vi "Run.vi"(8 "error in (no error)":errorcluster, 11 "Application in":refnum<class "Application.lvclass">) -> (0 "error out":errorcluster, 3 "Application out":refnum<class "Application.lvclass">)   [LabVIEW 2018, in "Application.lvclass"]
doc: "Este VI realiza a comunicação com as cãmeras através de uma estrutura de Fila. Possui uma máquina de estados que realiza o gerenciamento de cada informação que deve ser mandada para as câmeras e, também, é responsável por retornar o gráfico da última imagem obtida."
uses:
  Application.lvclass
  Application.lvclass/Application.ctl
  Instrument/Instrument.lvclass/Instrument.ctl
  State Machine/State Machine.lvclass/State Machine.ctl
  RxTx/RxTx.lvclass/RxTx.ctl
  CCDCamera/CCDCamera.lvclass/CCDCamera.ctl
  RxTXCamera/RxTxCamera.lvclass/RxTxCamera.ctl
  Construct String Header/Construct String Header.lvclass/Construct String Header.ctl
  RxTx/Write Message.vi
  RxTXCamera/Write Construct String Header.lvclass.vi
  RxTXCamera/Read Construct String Header.lvclass.vi
  Construct String Header/Write Header Contents.vi
  CCDCamera/CCDCamera.lvclass
  C:/Users/Cliente/Desktop/Software Echarpe/Instrument/Instrument.lvclass
  RxTXCamera/RxTxCamera.lvclass
  C:/Users/Cliente/Desktop/Software Echarpe/RxTx/RxTx.lvclass
  Construct String Header/Make string.vi
  State Machine/State Machine.lvclass
  Construct String Header/Construct String Header.lvclass
  Display Image/Display Image.lvclass
  Instrument/Instrument.lvclass
  RxTx/RxTx.lvclass
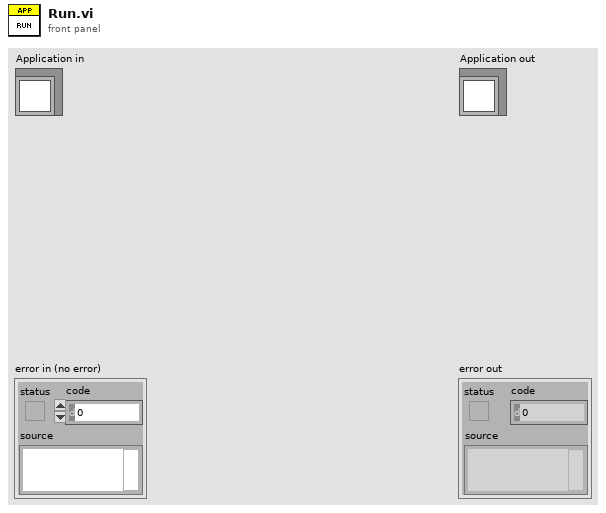
[diagram p1: front panel]
types:
  T1 = cluster{"Currently Temperature":dbl, "Last Image":string, "% Acquired":dbl, "Initilizarion":bool, "Exposing":bool, "Temperature Status":string, "X length":dbl, "Y length":dbl, "Min Temperature":dbl, "Max Temperature":dbl}
  T2 = cluster{"FILENAME":string[], "OBSERVER":string[], "PROGRID":string[], "OBJECT":string[], "NIGHTDIR":string[], "CHANNEL":string[], "INSTRUME":string[], "NEXPSEQ":string[], "SEQINDEX":string[], "OBSTYPE":string[], "READMOD":string[], "SHUTTER":string[], "OPENSHT":string[], "CLOSESHT":string[], "GAIN":string[], "GAINERR ":string[], "RDNOISE":string[], "RNOISERR":string[], "SKYFIBER":string[], "CALFIBER":string[], "UTDATE":string[], "LOCTIME":string[], "MJD":string[], "OBSLON":string[], "OBSLAT":string[], "OBSALT":string[], "EXPTIME":string[], "TELRA":string[], "TELDEC":string[], "RA":string[], "DEC":string[], "RA_DEG":string[], "DEC_DEG":string[], "EPOCH":string[], "HA":string[], "HAD":string[], "AIRMASS":string[], "AMSTART":string[], "AMEND":string[], "XOFFSET":string[], "YOFFSET":string[], "PA":string[], "CAMFOC":string[], "TELFOC":string[], "TCSUT":string[], "MOONDIST":string[], "MOONALT":string[], "MONNPHAS":string[], "ADC":string[], "ADCSPPED":string[], "CALMIRR":string[], "GUIDING":string[], "GUIDTEXP":string[], "GUIDFREQ":string[], "GUIDOBJX":string[], "GUIDOBJY":string[], "AVGYCORR":string[], "AVGXCORR":string[], "GFOCUS":string[], "THARLAMP":string[], "HALLAMP":string[], "AGITATOR":string[], "THARMIRR":string[], "DSTATUS":string[], "DTEMP":string[], "DHUM":string[], "DLAMP":string[], "DFLAT":string[], "TEMPEXT":string[], "PRESSURE":string[], "HUMIDITY":string[], "WINDDIR":string[], "WSPEED":string[], "TCSST":string[], "DPOS":string[]}
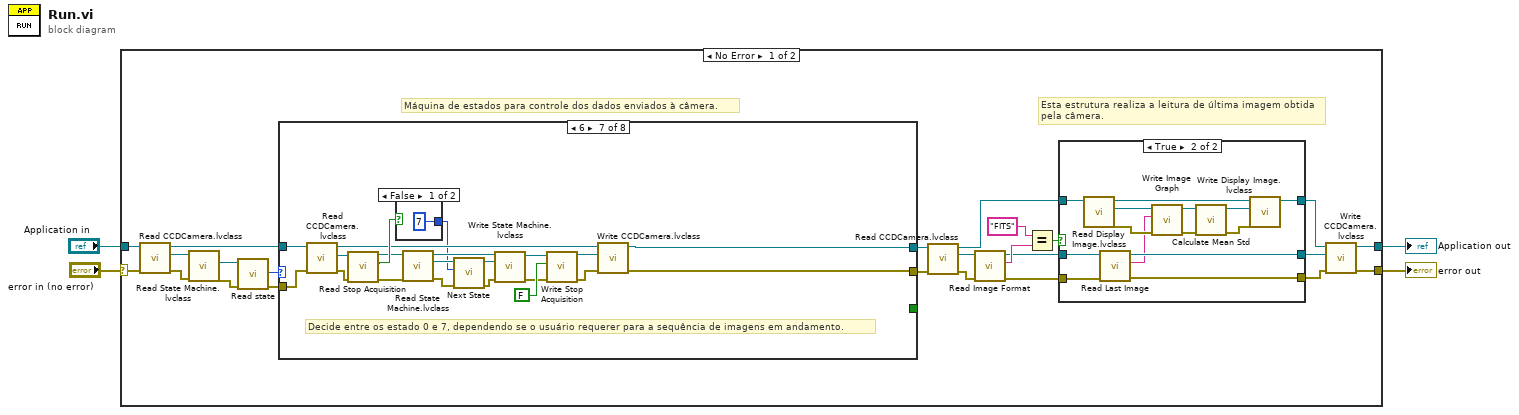
[diagram p0: block diagram]
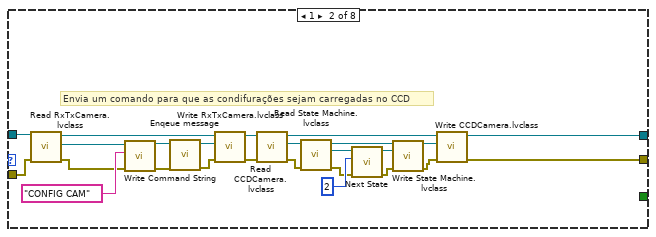
[diagram p3: hidden frame]
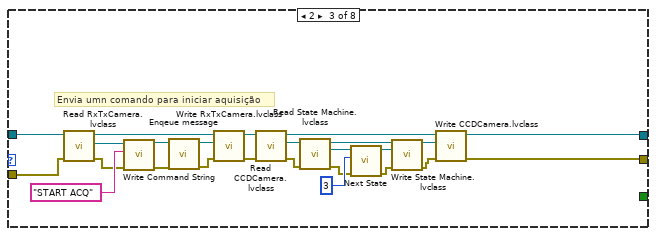
[diagram p4: hidden frame]
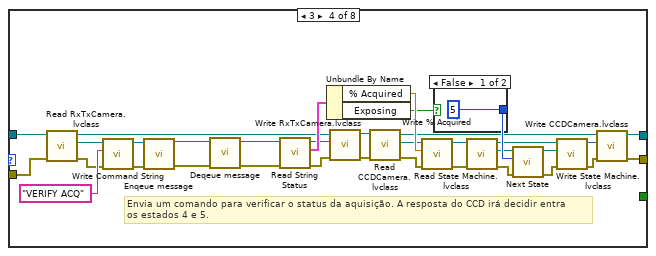
[diagram p5: hidden frame]
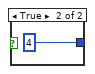
[diagram p6: hidden frame]
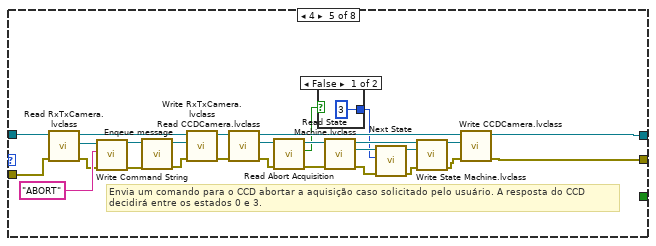
[diagram p7: hidden frame]
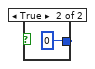
[diagram p8: hidden frame]
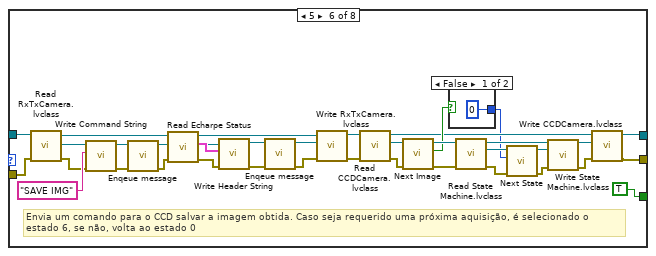
[diagram p9: hidden frame]
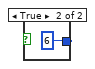
[diagram p10: hidden frame]
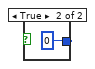
[diagram p11: hidden frame]
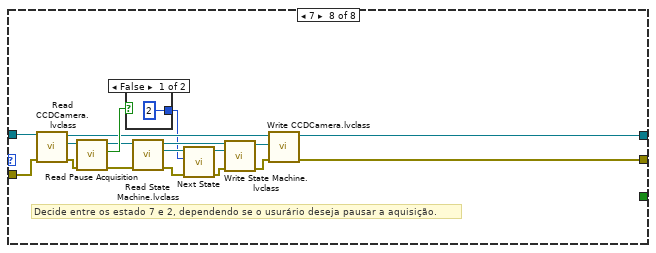
[diagram p12: hidden frame]
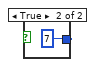
[diagram p13: hidden frame]
diagram:
  n1 = case shown="No Error" "error in (no error)" {
    selector: "error in (no error)" -> [w27 w246]
    tunnel: [w21 w246] -> w3
    tunnel: [w22 w245] -> w1
    tunnel: "Application in" -> [w28 w245]
    frame No Error {
      # "Esta estrutura realiza a leitura de última imagem obtida\npela câmera."
      # "Máquina de estados para controle dos dados enviados à câmera."
      n2 = call "Read CCDCamera.lvclass.vi"("error in (no error)"=w27, "Application in"=w28) -> ("error out"=w25:errorcluster, "CCDCamera.lvclass"=w26:refnum<class "CCDCamera.lvclass">, "Application out"=w7:refnum<class "Application.lvclass">)  [unwired: 7 in]
      n3 = call "Read State Machine.lvclass.vi"("error in (no error)"=w25, "Instrument in"=w26) -> ("error out"=w23:errorcluster, "State Machine.lvclass"=w24:refnum<class "State Machine.lvclass">)  [unwired: 7 in, 1 out]
      n4 = call "Read state.vi"("error in (no error)"=w23, "State Machine in"=w24) -> ("error out"=w6:errorcluster, "state"=w5:u32)  [unwired: 7 in, 1 out]
      n5 = case shown="6" w5 {
        tunnel: w6 -> [w29 w55 w58 w113 w125 w154 w187 w210]
        tunnel: w7 -> [w30 w54 w59 w114 w126 w155 w188 w211]
        tunnel: [w30 w32 w57 w82 w118 w168 w185 w209] -> w8
        tunnel: [w29 w31 w56 w81 w117 w167 w186 w208] -> w9
        tunnel: [_ _ _ _ _ TRUE _ _] -> _
        frame 0, Default {
        }
        frame 1 {
          # "Envia um comando para que as condifurações sejam carregadas no CCD"
          n6 = call "Read RxTxCamera.lvclass.vi"("error in (no error)"=w55, "Application in"=w54) -> ("error out"=w46:errorcluster, "RxTxCamera.lvclass"=w48:refnum<class "RxTxCamera.lvclass">, "Application out"=w52:refnum<class "Application.lvclass">)  [unwired: 7 in]
          n7 = call "Write Command String.vi"("error in (no error)"=w46, "Command String"="CONFIG CAM", "RxTxCamera in"=w48) -> ("error out"=w51:errorcluster, "RxTxCamera out"=w50:refnum<class "RxTxCamera.lvclass">)  [unwired: 7 in]
          n8 = call "Enqeue message.vi"("error in (no error)"=w51, "RxTx in"=w50) -> ("error out"=w53:errorcluster, "RxTx out"=w49:refnum<class "RxTxCamera.lvclass">)  [unwired: 8 in]
          n9 = call "Write RxTxCamera.lvclass.vi"("error in (no error)"=w53, "RxTxCamera.lvclass"=w49, "Application in"=w52) -> ("error out"=w45:errorcluster, "Application out"=w44:refnum<class "Application.lvclass">)  [unwired: 7 in]
          n10 = call "Read CCDCamera.lvclass.vi"("error in (no error)"=w45, "Application in"=w44) -> ("error out"=w43:errorcluster, "CCDCamera.lvclass"=w42:refnum<class "CCDCamera.lvclass">, "Application out"=w35:refnum<class "Application.lvclass">)  [unwired: 7 in]
          n11 = call "Read State Machine.lvclass.vi"("error in (no error)"=w43, "Instrument in"=w42) -> ("error out"=w40:errorcluster, "State Machine.lvclass"=w39:refnum<class "State Machine.lvclass">, "Instrument out"=w36:refnum<class "CCDCamera.lvclass">)  [unwired: 7 in]
          n12 = call "Next State.vi"("error in (no error)"=w40, "New_State"=u32 2, "State Machine in"=w39) -> ("error out"=w38:errorcluster, "State Machine out"=w37:refnum<class "State Machine.lvclass">)  [unwired: 7 in]
          n13 = call "Write State Machine.lvclass.vi"("error in (no error)"=w38, "State Machine.lvclass"=w37, "Instrument in"=w36) -> ("error out"=w34:errorcluster, "Instrument out"=w33:refnum<class "CCDCamera.lvclass">)  [unwired: 7 in]
          n14 = call "Write CCDCamera.lvclass.vi"("error in (no error)"=w34, "CCDCamera.lvclass"=w33, "Application in"=w35) -> ("error out"=w31:errorcluster, "Application out"=w32:refnum<class "Application.lvclass">)  [unwired: 7 in]
        }
        frame 2 {
          # "Envia umn comando para iniciar aquisição"
          n15 = call "Read RxTxCamera.lvclass.vi"("error in (no error)"=w58, "Application in"=w59) -> ("error out"=w73:errorcluster, "RxTxCamera.lvclass"=w75:refnum<class "RxTxCamera.lvclass">, "Application out"=w79:refnum<class "Application.lvclass">)  [unwired: 7 in]
          n16 = call "Write Command String.vi"("error in (no error)"=w73, "Command String"="START ACQ", "RxTxCamera in"=w75) -> ("error out"=w78:errorcluster, "RxTxCamera out"=w77:refnum<class "RxTxCamera.lvclass">)  [unwired: 7 in]
          n17 = call "Enqeue message.vi"("error in (no error)"=w78, "RxTx in"=w77) -> ("error out"=w80:errorcluster, "RxTx out"=w76:refnum<class "RxTxCamera.lvclass">)  [unwired: 8 in]
          n18 = call "Write RxTxCamera.lvclass.vi"("error in (no error)"=w80, "RxTxCamera.lvclass"=w76, "Application in"=w79) -> ("error out"=w72:errorcluster, "Application out"=w71:refnum<class "Application.lvclass">)  [unwired: 7 in]
          n19 = call "Read CCDCamera.lvclass.vi"("error in (no error)"=w72, "Application in"=w71) -> ("error out"=w70:errorcluster, "CCDCamera.lvclass"=w69:refnum<class "CCDCamera.lvclass">, "Application out"=w62:refnum<class "Application.lvclass">)  [unwired: 7 in]
          n20 = call "Read State Machine.lvclass.vi"("error in (no error)"=w70, "Instrument in"=w69) -> ("error out"=w67:errorcluster, "State Machine.lvclass"=w66:refnum<class "State Machine.lvclass">, "Instrument out"=w63:refnum<class "CCDCamera.lvclass">)  [unwired: 7 in]
          n21 = call "Next State.vi"("error in (no error)"=w67, "New_State"=u32 3, "State Machine in"=w66) -> ("error out"=w65:errorcluster, "State Machine out"=w64:refnum<class "State Machine.lvclass">)  [unwired: 7 in]
          n22 = call "Write State Machine.lvclass.vi"("error in (no error)"=w65, "State Machine.lvclass"=w64, "Instrument in"=w63) -> ("error out"=w61:errorcluster, "Instrument out"=w60:refnum<class "CCDCamera.lvclass">)  [unwired: 7 in]
          n23 = call "Write CCDCamera.lvclass.vi"("error in (no error)"=w61, "CCDCamera.lvclass"=w60, "Application in"=w62) -> ("error out"=w56:errorcluster, "Application out"=w57:refnum<class "Application.lvclass">)  [unwired: 7 in]
        }
        frame 3 {
          # "Envia um comando para verificar o status da aquisição. A resposta do CCD irá decidir entra\nos estados 4 e 5."
          n24 = call "Read RxTxCamera.lvclass.vi"("error in (no error)"=w113, "Application in"=w114) -> ("error out"=w106:errorcluster, "RxTxCamera.lvclass"=w107:refnum<class "RxTxCamera.lvclass">, "Application out"=w100:refnum<class "Application.lvclass">)  [unwired: 7 in]
          n25 = call "Write Command String.vi"("error in (no error)"=w106, "Command String"="VERIFY ACQ", "RxTxCamera in"=w107) -> ("error out"=w109:errorcluster, "RxTxCamera out"=w105:refnum<class "RxTxCamera.lvclass">)  [unwired: 7 in]
          n26 = call "Enqeue message.vi"("error in (no error)"=w109, "RxTx in"=w105) -> ("error out"=w104:errorcluster, "RxTx out"=w103:refnum<class "RxTxCamera.lvclass">)  [unwired: 8 in]
          n27 = call "Deqeue message.vi"("error in (no error)"=w104, "RxTx in"=w103) -> ("error out"=w112:errorcluster, "RxTx out"=w111:refnum<class "RxTxCamera.lvclass">)  [unwired: 8 in]
          n28 = call "Read String Status.vi"("error in (no error)"=w112, "RxTxCamera in"=w111) -> ("error out"=w102:errorcluster, "Camera Status"=w110:T1, "RxTxCamera out"=w101:refnum<class "RxTxCamera.lvclass">)  [unwired: 7 in]
          n29 = Unbundle By Name(w110) -> ("% Acquired"=w97:dbl, "Exposing"=w90:bool)
          n30 = call "Write RxTxCamera.lvclass.vi"("error in (no error)"=w102, "RxTxCamera.lvclass"=w101, "Application in"=w100) -> ("error out"=w99:errorcluster, "Application out"=w98:refnum<class "Application.lvclass">)  [unwired: 7 in]
          n31 = call "Read CCDCamera.lvclass.vi"("error in (no error)"=w99, "Application in"=w98) -> ("error out"=w95:errorcluster, "CCDCamera.lvclass"=w96:refnum<class "CCDCamera.lvclass">, "Application out"=w83:refnum<class "Application.lvclass">)  [unwired: 7 in]
          n32 = call "Write % Acquired.vi"("error in (no error)"=w95, "% Acquired"=w97, "CCDCamera in"=w96) -> ("error out"=w92:errorcluster, "CCDCamera out"=w91:refnum<class "CCDCamera.lvclass">)  [unwired: 7 in]
          n33 = case shown="False" w90 {
            tunnel: [u32 5 ("New_State") u32 4 ("New_State")] -> w89
            frame False {
            }
            frame True {
            }
          }
          n34 = call "Read State Machine.lvclass.vi"("error in (no error)"=w92, "Instrument in"=w91) -> ("error out"=w94:errorcluster, "State Machine.lvclass"=w88:refnum<class "State Machine.lvclass">, "Instrument out"=w86:refnum<class "CCDCamera.lvclass">)  [unwired: 7 in]
          n35 = call "Next State.vi"("error in (no error)"=w94, "New_State"=w89, "State Machine in"=w88) -> ("error out"=w93:errorcluster, "State Machine out"=w87:refnum<class "State Machine.lvclass">)  [unwired: 7 in]
          n36 = call "Write State Machine.lvclass.vi"("error in (no error)"=w93, "State Machine.lvclass"=w87, "Instrument in"=w86) -> ("error out"=w85:errorcluster, "Instrument out"=w84:refnum<class "CCDCamera.lvclass">)  [unwired: 7 in]
          n37 = call "Write CCDCamera.lvclass.vi"("error in (no error)"=w85, "CCDCamera.lvclass"=w84, "Application in"=w83) -> ("error out"=w81:errorcluster, "Application out"=w82:refnum<class "Application.lvclass">)  [unwired: 7 in]
        }
        frame 4 {
          # "Envia um comando para o CCD abortar a aquisição caso solicitado pelo usuário. A resposta do CCD\ndecidirá entre os estados 0 e 3."
          n38 = call "Read RxTxCamera.lvclass.vi"("error in (no error)"=w125, "Application in"=w126) -> ("error out"=w137:errorcluster, "RxTxCamera.lvclass"=w139:refnum<class "RxTxCamera.lvclass">, "Application out"=w143:refnum<class "Application.lvclass">)  [unwired: 7 in]
          n39 = call "Write Command String.vi"("error in (no error)"=w137, "Command String"="ABORT", "RxTxCamera in"=w139) -> ("error out"=w142:errorcluster, "RxTxCamera out"=w141:refnum<class "RxTxCamera.lvclass">)  [unwired: 7 in]
          n40 = call "Enqeue message.vi"("error in (no error)"=w142, "RxTx in"=w141) -> ("error out"=w144:errorcluster, "RxTx out"=w140:refnum<class "RxTxCamera.lvclass">)  [unwired: 8 in]
          n41 = call "Write RxTxCamera.lvclass.vi"("error in (no error)"=w144, "RxTxCamera.lvclass"=w140, "Application in"=w143) -> ("error out"=w136:errorcluster, "Application out"=w135:refnum<class "Application.lvclass">)  [unwired: 7 in]
          n42 = call "Read CCDCamera.lvclass.vi"("error in (no error)"=w136, "Application in"=w135) -> ("error out"=w123:errorcluster, "CCDCamera.lvclass"=w124:refnum<class "CCDCamera.lvclass">, "Application out"=w129:refnum<class "Application.lvclass">)  [unwired: 7 in]
          n43 = call "Read Abort Acquisition.vi"("error in (no error)"=w123, "CCDCamera in"=w124) -> ("error out"=w122:errorcluster, "Abort Acquisition"=w120:bool, "CCDCamera out"=w121:refnum<class "CCDCamera.lvclass">)  [unwired: 7 in]
          n44 = case shown="False" w120 {
            tunnel: [u32 3 ("New_State") u32 0 ("New_State")] -> w119
            frame False {
            }
            frame True {
            }
          }
          n45 = call "Read State Machine.lvclass.vi"("error in (no error)"=w122, "Instrument in"=w121) -> ("error out"=w134:errorcluster, "State Machine.lvclass"=w133:refnum<class "State Machine.lvclass">, "Instrument out"=w130:refnum<class "CCDCamera.lvclass">)  [unwired: 7 in]
          n46 = call "Next State.vi"("error in (no error)"=w134, "New_State"=w119, "State Machine in"=w133) -> ("error out"=w132:errorcluster, "State Machine out"=w131:refnum<class "State Machine.lvclass">)  [unwired: 7 in]
          n47 = call "Write State Machine.lvclass.vi"("error in (no error)"=w132, "State Machine.lvclass"=w131, "Instrument in"=w130) -> ("error out"=w128:errorcluster, "Instrument out"=w127:refnum<class "CCDCamera.lvclass">)  [unwired: 7 in]
          n48 = call "Write CCDCamera.lvclass.vi"("error in (no error)"=w128, "CCDCamera.lvclass"=w127, "Application in"=w129) -> ("error out"=w117:errorcluster, "Application out"=w118:refnum<class "Application.lvclass">)  [unwired: 7 in]
        }
        frame 5 {
          # "Envia um comando para o CCD salvar a imagem obtida. Caso seja requerido uma próxima aquisição, é selecionado o \nestado 6, se não, volta ao estado 0"
          n49 = call "Read RxTxCamera.lvclass.vi"("error in (no error)"=w154, "Application in"=w155) -> ("error out"=w152:errorcluster, "RxTxCamera.lvclass"=w151:refnum<class "RxTxCamera.lvclass">, "Application out"=w159:refnum<class "Application.lvclass">)  [unwired: 7 in]
          n50 = call "Write Command String.vi"("error in (no error)"=w152, "Command String"="SAVE IMG", "RxTxCamera in"=w151) -> ("error out"=w150:errorcluster, "RxTxCamera out"=w148:refnum<class "RxTxCamera.lvclass">)  [unwired: 7 in]
          n51 = call "Enqeue message.vi"("error in (no error)"=w150, "RxTx in"=w148) -> ("error out"=w149:errorcluster, "RxTx out"=w147:refnum<class "RxTxCamera.lvclass">)  [unwired: 8 in]
          n52 = call "Read Echarpe Status.vi"("error in (no error)"=w149, "Application in"=w159) -> ("error out"=w162:errorcluster, "Header Contents out"=w161:T2, "Application out"=w160:refnum<class "Application.lvclass">)  [unwired: 7 in]
          n53 = call "Write Header String.vi"("error in (no error)"=w162, "Header Contents"=w161, "RxTxCamera in"=w147) -> ("error out"=w163:errorcluster, "RxTxCamera out"=w164:refnum<class "RxTxCamera.lvclass">)  [unwired: 7 in]
          n54 = call "Enqeue message.vi"("error in (no error)"=w163, "RxTx in"=w164) -> ("error out"=w165:errorcluster, "RxTx out"=w166:refnum<class "RxTxCamera.lvclass">)  [unwired: 8 in]
          n55 = call "Write RxTxCamera.lvclass.vi"("error in (no error)"=w165, "RxTxCamera.lvclass"=w166, "Application in"=w160) -> ("error out"=w157:errorcluster, "Application out"=w156:refnum<class "Application.lvclass">)  [unwired: 7 in]
          n56 = call "Read CCDCamera.lvclass.vi"("error in (no error)"=w157, "Application in"=w156) -> ("error out"=w178:errorcluster, "CCDCamera.lvclass"=w179:refnum<class "CCDCamera.lvclass">, "Application out"=w172:refnum<class "Application.lvclass">)  [unwired: 7 in]
          n57 = call "Next Image"("error in (no error)"=w178, "CCDCamera in"=w179) -> ("error out"=w182:errorcluster, "Next Image ?"=w180:bool, "CCDCamera out"=w181:refnum<class "CCDCamera.lvclass">)  [unwired: 7 in]
          n58 = case shown="False" w180 {
            tunnel: [u32 0 ("New_State") u32 6 ("New_State")] -> w169
            frame False {
            }
            frame True {
            }
          }
          n59 = call "Read State Machine.lvclass.vi"("error in (no error)"=w182, "Instrument in"=w181) -> ("error out"=w177:errorcluster, "State Machine.lvclass"=w176:refnum<class "State Machine.lvclass">, "Instrument out"=w173:refnum<class "CCDCamera.lvclass">)  [unwired: 7 in]
          n60 = call "Next State.vi"("error in (no error)"=w177, "New_State"=w169, "State Machine in"=w176) -> ("error out"=w175:errorcluster, "State Machine out"=w174:refnum<class "State Machine.lvclass">)  [unwired: 7 in]
          n61 = call "Write State Machine.lvclass.vi"("error in (no error)"=w175, "State Machine.lvclass"=w174, "Instrument in"=w173) -> ("error out"=w171:errorcluster, "Instrument out"=w170:refnum<class "CCDCamera.lvclass">)  [unwired: 7 in]
          n62 = call "Write CCDCamera.lvclass.vi"("error in (no error)"=w171, "CCDCamera.lvclass"=w170, "Application in"=w172) -> ("error out"=w167:errorcluster, "Application out"=w168:refnum<class "Application.lvclass">)  [unwired: 7 in]
        }
        frame 6 {
          # "Decide entre os estado 0 e 7, dependendo se o usuário requerer para a sequência de imagens em andamento."
          n63 = call "Read CCDCamera.lvclass.vi"("error in (no error)"=w187, "Application in"=w188) -> ("error out"=w197:errorcluster, "CCDCamera.lvclass"=w196:refnum<class "CCDCamera.lvclass">, "Application out"=w190:refnum<class "Application.lvclass">)  [unwired: 7 in]
          n64 = call "Read Stop Acquisition.vi"("error in (no error)"=w197, "CCDCamera in"=w196) -> ("error out"=w198:errorcluster, "Stop Acquisition"=w200:bool, "CCDCamera out"=w199:refnum<class "CCDCamera.lvclass">)  [unwired: 7 in]
          n65 = case shown="False" w200 {
            tunnel: [u32 7 ("New_State") u32 0 ("New_State")] -> w189
            frame False {
            }
            frame True {
            }
          }
          n66 = call "Read State Machine.lvclass.vi"("error in (no error)"=w198, "Instrument in"=w199) -> ("error out"=w195:errorcluster, "State Machine.lvclass"=w194:refnum<class "State Machine.lvclass">, "Instrument out"=w191:refnum<class "CCDCamera.lvclass">)  [unwired: 7 in]
          n67 = call "Next State.vi"("error in (no error)"=w195, "New_State"=w189, "State Machine in"=w194) -> ("error out"=w193:errorcluster, "State Machine out"=w192:refnum<class "State Machine.lvclass">)  [unwired: 7 in]
          n68 = call "Write State Machine.lvclass.vi"("error in (no error)"=w193, "State Machine.lvclass"=w192, "Instrument in"=w191) -> ("error out"=w201:errorcluster, "Instrument out"=w202:refnum<class "CCDCamera.lvclass">)  [unwired: 7 in]
          n69 = call "Write Stop Acquisition.vi"("error in (no error)"=w201, "Stop Acquisition"=FALSE, "CCDCamera in"=w202) -> ("error out"=w203:errorcluster, "CCDCamera out"=w204:refnum<class "CCDCamera.lvclass">)  [unwired: 7 in]
          n70 = call "Write CCDCamera.lvclass.vi"("error in (no error)"=w203, "CCDCamera.lvclass"=w204, "Application in"=w190) -> ("error out"=w186:errorcluster, "Application out"=w185:refnum<class "Application.lvclass">)  [unwired: 7 in]
        }
        frame 7 {
          # "Decide entre os estado 7 e 2, dependendo se o usurário deseja pausar a aquisição."
          n71 = call "Read CCDCamera.lvclass.vi"("error in (no error)"=w210, "Application in"=w211) -> ("error out"=w219:errorcluster, "CCDCamera.lvclass"=w220:refnum<class "CCDCamera.lvclass">, "Application out"=w213:refnum<class "Application.lvclass">)  [unwired: 7 in]
          n72 = call "Read Pause Acquisition.vi"("error in (no error)"=w219, "CCDCamera in"=w220) -> ("error out"=w221:errorcluster, "Pause Acquisition"=w223:bool, "CCDCamera out"=w222:refnum<class "CCDCamera.lvclass">)  [unwired: 7 in]
          n73 = case shown="False" w223 {
            tunnel: [u32 2 ("New_State") u32 7 ("New_State")] -> w212
            frame False {
            }
            frame True {
            }
          }
          n74 = call "Read State Machine.lvclass.vi"("error in (no error)"=w221, "Instrument in"=w222) -> ("error out"=w218:errorcluster, "State Machine.lvclass"=w217:refnum<class "State Machine.lvclass">, "Instrument out"=w214:refnum<class "CCDCamera.lvclass">)  [unwired: 7 in]
          n75 = call "Next State.vi"("error in (no error)"=w218, "New_State"=w212, "State Machine in"=w217) -> ("error out"=w216:errorcluster, "State Machine out"=w215:refnum<class "State Machine.lvclass">)  [unwired: 7 in]
          n76 = call "Write State Machine.lvclass.vi"("error in (no error)"=w216, "State Machine.lvclass"=w215, "Instrument in"=w214) -> ("error out"=w224:errorcluster, "Instrument out"=w225:refnum<class "CCDCamera.lvclass">)  [unwired: 7 in]
          n77 = call "Write CCDCamera.lvclass.vi"("error in (no error)"=w224, "CCDCamera.lvclass"=w225, "Application in"=w213) -> ("error out"=w208:errorcluster, "Application out"=w209:refnum<class "Application.lvclass">)  [unwired: 7 in]
        }
      }
      n78 = call "Read CCDCamera.lvclass.vi"("error in (no error)"=w9, "Application in"=w8) -> ("error out"=w12:errorcluster, "CCDCamera.lvclass"=w11:refnum<class "CCDCamera.lvclass">, "Application out"=w10:refnum<class "Application.lvclass">)  [unwired: 7 in]
      n79 = call "Read Image Format.vi"("error in (no error)"=w12, "CCDCamera in"=w11) -> ("error out"=w13:errorcluster, "Image Format"=w16:string, "CCDCamera out"=w14:refnum<class "CCDCamera.lvclass">)  [unwired: 7 in]
      n80 = Equal?(x="FITS", y=w16) -> (x = y?=w17:bool)
      n81 = case shown="True" w17 {
        tunnel: [w228 w237] -> w20
        tunnel: [w230 w236] -> w19
        tunnel: [w229 w235] -> w18
        tunnel: w13 -> [w229 w234]
        tunnel: w14 -> [w230 w233]
        tunnel: w10 -> [w228 w231]
        frame False {
        }
        frame True {
          n82 = call "Read Display Image.lvclass.vi"("Application in"=w231) -> ("error out"=w243:errorcluster, "Display Image.lvclass"=w244:refnum<class "Display Image.lvclass">, "Application out"=w238:refnum<class "Application.lvclass">)  [unwired: 8 in]
          n83 = call "Read Last Image.vi"("error in (no error)"=w234, "CCDCamera in"=w233) -> ("error out"=w235:errorcluster, "Last Image Path"=w232:string, "CCDCamera out"=w236:refnum<class "CCDCamera.lvclass">)  [unwired: 6 in, 1 out]
          n84 = call "Write Image Graph.vi"("error in (no error)"=w243, "file path"=w232, "Display Image in"=w244) -> ("error out"=w242:errorcluster, "Display Image out"=w241:refnum<class "Display Image.lvclass">)  [unwired: 7 in]
          n85 = call "Calculate Mean Std.vi"("error in (no error)"=w242, "Display Image in"=w241) -> ("error out"=w240:errorcluster, "Display Image out"=w239:refnum<class "Display Image.lvclass">)  [unwired: 8 in]
          n86 = call "Write Display Image.lvclass.vi"("error in (no error)"=w240, "Display Image.lvclass"=w239, "Application in"=w238) -> ("Application out"=w237:refnum<class "Application.lvclass">)  [unwired: 7 in, 1 out]
        }
      }
      n87 = call "Write CCDCamera.lvclass.vi"("error in (no error)"=w18, "CCDCamera.lvclass"=w19, "Application in"=w20) -> ("error out"=w21:errorcluster, "Application out"=w22:refnum<class "Application.lvclass">)  [unwired: 7 in]
    }
    frame Error {
    }
  }
  "error out" <- w3
  "Application out" <- w1
